vi "Serialize Low Level Protocol Packet.vi"(0 "tagged llp packet":T1={"tag"={"timestamp"={"valid"=FALSE, "count"=0.0, "id"=enum."SI0 LLP", "metadata"=0}, "size"={"bytes"=0.0, "valid"=FALSE}}, "llp packet"={"header"={"word count"=0, "ecc"=0.0, "vcx"=0.0, "data type"=0.0, "vc"=0.0}, "header valid"=FALSE, "payload"={"end of payload"=FALSE, "end of payload index"=0.0, "payload data"=[0, 0, 0, 0]}, "payload valid"=FALSE, "footer"={"crc"=0}, "footer valid"=FALSE, "end of packet"=FALSE}}, 1 "reset":bool, 2 "flush":bool, 9 "input valid":bool, 11 "count packet size":bool, 12 "ready for output":bool=TRUE) -> (3 "flush complete":bool, 4 "serialized data":u8[](array[numeric]), 6 "valid bytes":fxp<+,4,4>, 8 "in reset":bool, 10 "output valid":bool, 14 "ready for input":bool, 15 "unread data":bool)   [LabVIEW 2020, in "GettingStarted_Acq_Tap_148X_FPGA.lvlib"]
uses:
  GettingStarted_Acq_Tap_148X_FPGA.lvlib
  <instrlib>/FlexRIO/CSI-2/v2/FPGA/Types/Tagged LLP Packet.ctl
  <instrlib>/FlexRIO/CSI-2/v2/FPGA/Types/FPGA LLP Packet Tag.ctl
  <instrlib>/FlexRIO/CSI-2/v2/FPGA/Types/FPGA LLP Packet Timestamp.ctl
  <instrlib>/FlexRIO/CSI-2/v2/FPGA/Types/Timestamp ID.ctl
  <instrlib>/FlexRIO/CSI-2/v2/FPGA/Types/FPGA LLP Packet Size.ctl
  <instrlib>/FlexRIO/CSI-2/v2/FPGA/Types/LLP Packet.ctl
  <instrlib>/FlexRIO/CSI-2/v2/FPGA/Types/LLP Packet Header.ctl
  <instrlib>/FlexRIO/CSI-2/v2/FPGA/Types/LLP Packet Payload.ctl
  <instrlib>/FlexRIO/CSI-2/v2/FPGA/Types/LLP Packet Footer.ctl
  ea058fa1-ed7a-440f-aab2-62066a9aa946.vi
  5b316473-bbfc-468e-b692-e536612e766d.vi
  <instrlib>/FlexRIO/CSI-2/v2/FPGA/NI CSI-2 API FPGA v2.lvlib
  <instrlib>/_niInstr/Basic Elements/v1/FPGA/niInstr Basic Elements v1 FPGA.lvlib
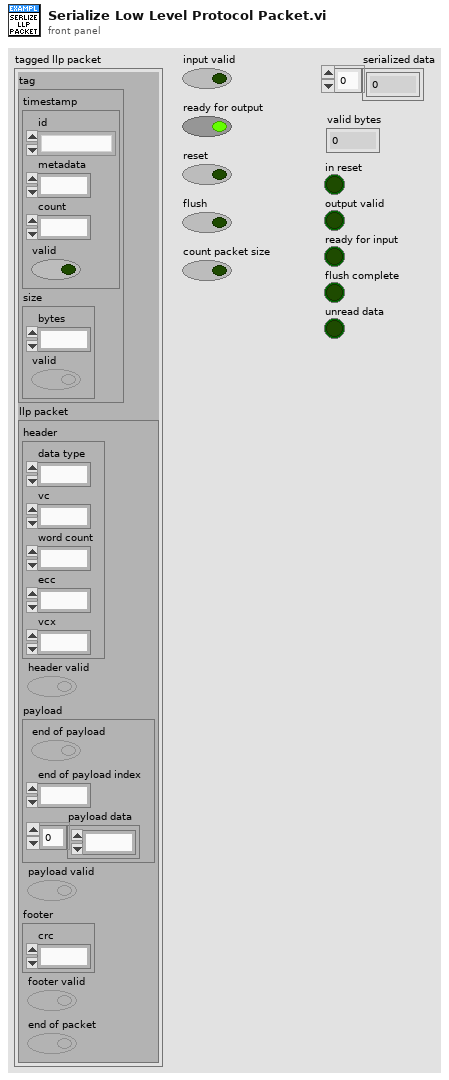
[diagram p1: front panel]
types:
  T1 = typedef "NI CSI-2 API FPGA v2.lvlib/Tagged LLP Packet.ctl" = cluster{"tag":T2, "llp packet":T6}
  T2 = typedef "NI CSI-2 API FPGA v2.lvlib/FPGA LLP Packet Tag.ctl" = cluster{"timestamp":T3, "size":T5}
  T3 = typedef "NI CSI-2 API FPGA v2.lvlib/FPGA LLP Packet Timestamp.ctl" = cluster{"valid":bool, "count":fxp<+,50,50>, "id":T4, "metadata":u8}
  T4 = typedef "NI CSI-2 API FPGA v2.lvlib/Timestamp ID.ctl" = enum8{"SI0 LLP", "SI1 LLP", "SI2 LLP", "SI3 LLP", "SI4 LLP", "SI5 LLP", "SI6 LLP", "SI7 LLP", "SO0 LLP", "SO1 LLP", "SO2 LLP", "SO3 LLP", "SO4 LLP", "SO5 LLP", "SO6 LLP", "SO7 LLP", "Ser0 GPIO Bank", "Ser1 GPIO Bank", "Ser2 GPIO Bank", "Ser3 GPIO Bank", "Ser4 GPIO Bank", "Ser5 GPIO Bank", "Ser6 GPIO Bank", "Ser7 GPIO Bank", "Des0 GPIO Bank", "Des1 GPIO Bank", "Des2 GPIO Bank", "Des3 GPIO Bank", "Des4 GPIO Bank", "Des5 GPIO Bank", "Des6 GPIO Bank", "Des7 GPIO Bank", "User0", "User1", "User2", "User3", "User4", "User5", "User6", "User7", "User8", "User9", "User10", "User11", "User12", "User13", "User14", "User15", "User16", "User17", "User18", "User19", "User20", "User21", "User22", "User23", "User24", "User25", "User26", "User27", "User28", "User29", "User30", "User31"}
  T5 = typedef "NI CSI-2 API FPGA v2.lvlib/FPGA LLP Packet Size.ctl" = cluster{"bytes":fxp<+,17,17>, "valid":bool}
  T6 = typedef "NI CSI-2 API FPGA v2.lvlib/LLP Packet.ctl" = cluster{"header":T7, "header valid":bool, "payload":T8, "payload valid":bool, "footer":T9, "footer valid":bool, "end of packet":bool}
  T7 = typedef "NI CSI-2 API FPGA v2.lvlib/LLP Packet Header.ctl" = cluster{"word count":u16, "ecc":fxp<+,6,6>, "vcx":fxp<+,2,2>, "data type":fxp<+,6,6>, "vc":fxp<+,2,2>}
  T8 = typedef "NI CSI-2 API FPGA v2.lvlib/LLP Packet Payload.ctl" = cluster{"end of payload":bool, "end of payload index":fxp<+,3,3>, "payload data":u8[]}
  T9 = typedef "NI CSI-2 API FPGA v2.lvlib/LLP Packet Footer.ctl" = cluster{"crc":u16}
  T10 = cluster{bool, "data out":u8[], "max":fxp<+,4,4>, bool, "output valid":bool}
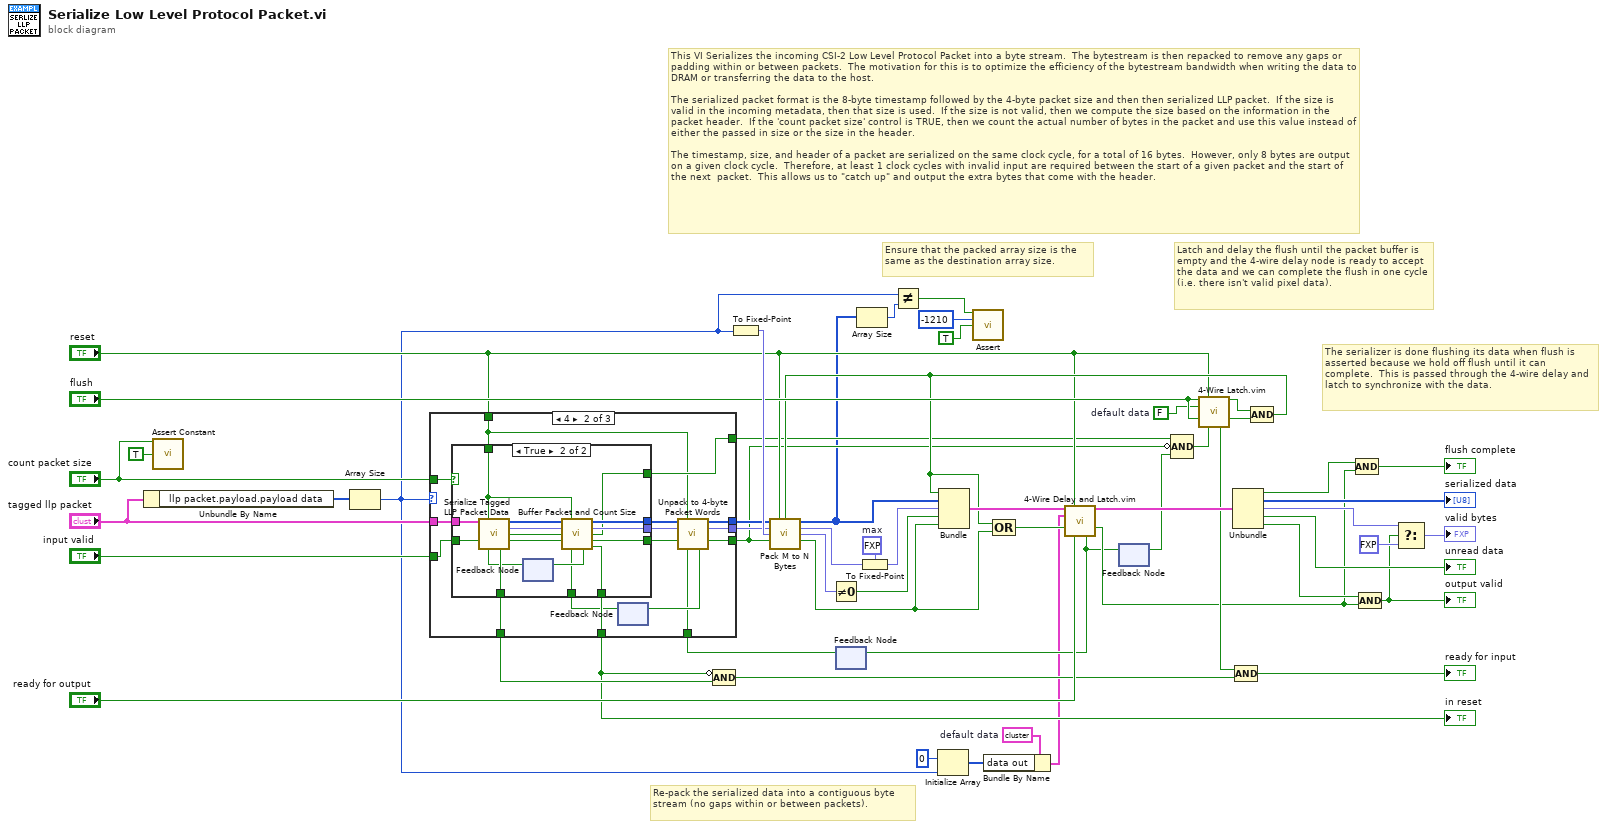
[diagram p0: block diagram]
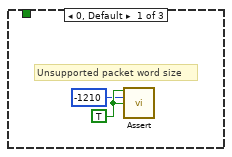
[diagram p2: hidden frame]
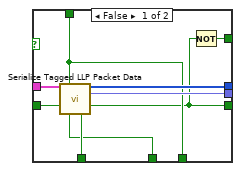
[diagram p3: hidden frame]
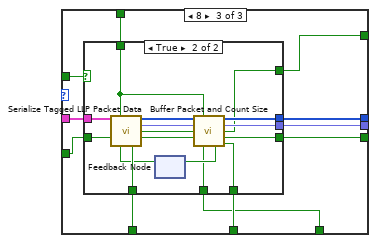
[diagram p4: hidden frame]
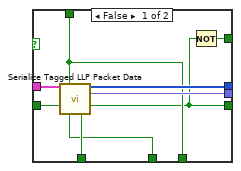
[diagram p5: hidden frame]
diagram:
  w5 = T10 {FALSE, "data out"=[], "max"=0.0, FALSE, "output valid"=FALSE}  # default data
  w6 = FALSE  # default data
  w48 = fxp<+,4,4> 8.0  # max
  # "This VI Serializes the incoming CSI-2 Low Level Protocol Packet into a byte stream.  The bytestream is then repacked to remove any gaps or padding within or between packets.  The motivation for this is to optimize the efficiency of the bytestream bandwidth when writing the data to DRAM or transferring the data to the host.\n\nThe serialized packet format is the 8-byte timestamp followed by the 4-byte packet size and then then serialized LLP packet.  If the size is valid in the incoming metadata, then that size is used.  If the size is not valid, then we compute the size based on the information in the packet header.  If the 'count packet size' control is TRUE, then we count the actual number of bytes in the packet and use this value instead of either the passed in size or the size in the header.\n\nThe timestamp, size, and header of a packet are serialized on the same clock cycle, for a total of 16 bytes.  However, only 8 bytes are output on a given clock cycle.  Therefore, at least 1 clock cycles with invalid input are required between the start of a given packet and the start of the next  packet.  This allows us to \"catch up\" and output the extra bytes that come with the header."
  # "Latch and delay the flush until the packet buffer is empty and the 4-wire delay node is ready to accept the data and we can complete the flush in one cycle (i.e. there isn't valid pixel data)."
  # "The serializer is done flushing its data when flush is asserted because we hold off flush until it can complete.  This is passed through the 4-wire delay and latch to synchronize with the data."
  # "Ensure that the packed array size is the same as the destination array size."
  # "Re-pack the serialized data into a contiguous byte stream (no gaps within or between packets)."
  n1 = Unbundle By Name("tagged llp packet") -> ("llp packet.payload.payload data"=w7:u8[])
  n2 = call <instrlib>:"Assert Constant.vi"("constant terminal"="count packet size", "enable show error"=TRUE) -> ()  [unwired: 14 in]
  n3 = Array Size(array=w7) -> (size(s)=w3:i32)
  n4 = To Fixed-Point(number=w3) -> (fixed-point=w49:fxp<+,5,5>)  [unwired: 1 in]
  n5 = feedback #1() -> (w11:bool)  [unwired: 1 in]
  n6 = case shown="4" w3 {
    tunnel: "tagged llp packet" -> [_ w73 w109]
    tunnel: "input valid" -> [_ w72 w108]
    tunnel: "count packet size" -> [_ w71 w107]
    tunnel: [_ w70 w106] -> w18
    tunnel: [_ w69 w105] -> w16
    tunnel: "reset" -> [_ w61 w104]
    tunnel: [_ w68 w103] -> w14
    tunnel: [_ w66 w102] -> w13
    tunnel: [_ w65 w101] -> w12
    tunnel: w11 -> [_ w58 w100]
    tunnel: [_ w62 w99] -> w10
    frame 0, Default {
      w57 = TRUE ("enable show error")
      # "Unsupported packet word size"
      n7 = call <instrlib>:"Assert.vi"("assert"=w57, "error code"=-1210, "enable show error"=w57) -> ()  [unwired: 13 in]
    }
    frame 4 {
      n8 = feedback #2() -> (w59:bool)  [unwired: 1 in]
      n9 = case shown="True" w71 {
        tunnel: w73 -> [w82 w98]
        tunnel: w72 -> [w81 w97]
        tunnel: [w80 w96] -> w70
        tunnel: [w79 w88] -> w67
        tunnel: w61 -> [w76 w89]
        tunnel: [w78 w87] -> w64
        tunnel: [w75 w86] -> w63
        tunnel: w59 -> [w77 w85]
        tunnel: [w76 w83] -> w69
        tunnel: [w74 w84] -> w68
        frame False {
          n10 = call "Serialize Tagged LLP Packet Data.vi"("tagged llp packet"=w82, "reset"=w76, "input valid"=w81, "ready for output"=w77) -> ("serialized data"=w79:u8[], "valid bytes"=w78:fxp<+,4,4>, "output valid"=w75:bool, "ready for input"=w80:bool)  [unwired: 7 in, 1 out]
          n11 = Not(x=w75) -> (.not. x?=w74:bool)
        }
        frame True {
          n12 = feedback #3() -> (w91:bool)  [unwired: 1 in]
          n13 = call "Serialize Tagged LLP Packet Data.vi"("tagged llp packet"=w98, "reset"=w89, "input valid"=w97, "ready for output"=w91) -> ("serialized data"=w95:u8[], "valid bytes"=w94:fxp<+,4,4>, "end of packet"=w90:bool, "output valid"=w93:bool, "ready for input"=w96:bool)  [unwired: 7 in]
          n14 = call "Buffer Packet and Count Size.vi"("serialized data in"=w95, "reset"=w89, "valid bytes in"=w94, "end of packet"=w90, "input valid"=w93, "ready for output"=w85) -> ("serialized data out"=w88:u8[], "valid bytes out"=w87:fxp<+,4,4>, "empty"=w84:bool, "output valid"=w86:bool, "ready for input"=w92:bool, "in reset"=w83:bool)  [unwired: 4 in]
          n15 = feedback-in #3(w92) -> ()
        }
      }
      n16 = call "Unpack to 4-byte Packet Words.vi"("serialized data in"=w67, "reset"=w61, "valid bytes in"=w64, "input valid"=w63, "ready for output"=w58) -> ("serialized data out"=w66:u8[], "valid bytes out"=w65:fxp<+,3,3>, "output valid"=w62:bool, "ready for input"=w60:bool)  [unwired: 7 in]
      n17 = feedback-in #2(w60) -> ()
    }
    frame 8 {
      n18 = case shown="True" w107 {
        tunnel: w109 -> [w118 w134]
        tunnel: w108 -> [w117 w133]
        tunnel: [w116 w132] -> w106
        tunnel: [w115 w124] -> w102
        tunnel: w104 -> [w112 w125]
        tunnel: [w114 w123] -> w101
        tunnel: [w111 w122] -> w99
        tunnel: w100 -> [w113 w121]
        tunnel: [w112 w119] -> w105
        tunnel: [w110 w120] -> w103
        frame False {
          n19 = call "Serialize Tagged LLP Packet Data.vi"("tagged llp packet"=w118, "reset"=w112, "input valid"=w117, "ready for output"=w113) -> ("serialized data"=w115:u8[], "valid bytes"=w114:fxp<+,4,4>, "output valid"=w111:bool, "ready for input"=w116:bool)  [unwired: 7 in, 1 out]
          n20 = Not(x=w111) -> (.not. x?=w110:bool)
        }
        frame True {
          n21 = feedback #4() -> (w127:bool)  [unwired: 1 in]
          n22 = call "Serialize Tagged LLP Packet Data.vi"("tagged llp packet"=w134, "reset"=w125, "input valid"=w133, "ready for output"=w127) -> ("serialized data"=w131:u8[], "valid bytes"=w130:fxp<+,4,4>, "end of packet"=w126:bool, "output valid"=w129:bool, "ready for input"=w132:bool)  [unwired: 7 in]
          n23 = call "Buffer Packet and Count Size.vi"("serialized data in"=w131, "reset"=w125, "valid bytes in"=w130, "end of packet"=w126, "input valid"=w129, "ready for output"=w121) -> ("serialized data out"=w124:u8[], "valid bytes out"=w123:fxp<+,4,4>, "empty"=w120:bool, "output valid"=w122:bool, "ready for input"=w128:bool, "in reset"=w119:bool)  [unwired: 4 in]
          n24 = feedback-in #4(w128) -> ()
        }
      }
    }
  }
  "in reset" <- w16
  n25 = Compound Arithmetic op=AND(invert w16, w18) -> (w17:bool)
  n26 = Initialize Array(u8 0 ("element"), w3) -> (w4:u8[])
  n27 = Bundle By Name(cluster=w5, "data out"=w4) -> (w1:T10)
  n28 = feedback #5() -> (w37:bool)  [unwired: 1 in]
  n29 = Compound Arithmetic op=AND(w14, invert w10, w37) -> (w36:bool)
  n30 = call "4-Wire Latch.vim"("data in"="flush", "reset"="reset", "default data"=w6, "input valid"="flush", "ready for output"=w36) -> ("data out"=w47:bool, "output valid"=w46:bool, "ready for input"=w34:bool)  [unwired: 8 in]
  n31 = Compound Arithmetic op=AND(w34, w17) -> (→"ready for input":bool)
  n32 = Compound Arithmetic op=AND(w47, w46) -> (w28:bool)
  n33 = call <instrlib>:"Pack M to N Bytes.vi"("data in"=w13, "reset"="reset", "flush"=w28, "valid bytes in"=w12, "output size"=w49, "input valid"=w10) -> ("data out"=w9:u8[], "valid bytes out"=w54:fxp<+,5,5>, "unread bytes"=w55:fxp<+,4,4>, "output valid"=w25:bool)  [unwired: 4 in, 2 out]
  n34 = Not Equal To 0?(x=w55) -> (x != 0?=w40:bool)
  n35 = Array Size(array=w9) -> (size(s)=w53:i32)
  n36 = To Fixed-Point(fixed-point type=w48, number=w54) -> (fixed-point=w45:fxp<+,4,4>)
  n37 = Not Equal?(x=w3, y=w53) -> (x != y?=w50:bool)
  n38 = Bundle(w28, "data out"=w9, "max"=w45, w40, "output valid"=w25) -> (w44:T10)  [unwired: 1 in]
  n39 = call <instrlib>:"Assert.vi"("assert"=w50, "error code"=-1210, "enable show error"=TRUE) -> ()  [unwired: 13 in]
  n40 = Compound Arithmetic op=OR(w28, w25) -> (w29:bool)
  n41 = call "4-Wire Delay and Latch.vim"("data in"=w44, "reset"="reset", "default data"=w1, "input valid"=w29, "ready for output"="ready for output") -> ("data out"=w43:T10, "output valid"=w23:bool, "ready for input"=w21:bool)  [unwired: 8 in]
  n42 = feedback-in #1(w21) -> ()
  n43 = feedback-in #5(w21) -> ()
  n44 = Unbundle(w43) -> (w42:bool, "data out"=→"serialized data":u8[], "max"=w31:fxp<+,4,4>, →"unread data":bool, "output valid"=w24:bool)
  n45 = Compound Arithmetic op=AND(w42, w23) -> (→"flush complete":bool)
  n46 = Compound Arithmetic op=AND(w24, w23) -> (w22:bool)
  "output valid" <- w22
  n47 = Select(t=w31, s=w22, f=fxp<+,4,4> 0.0) -> (s? t:f=→"valid bytes":fxp<+,4,4>)
